vi "Orca Data Spooler Check TL Filename.vi"(0 "Path":path, 11 "Error In":errorcluster) -> (4 "Proof Path":path, 15 "Error Out":errorcluster)   [LabVIEW 2020]
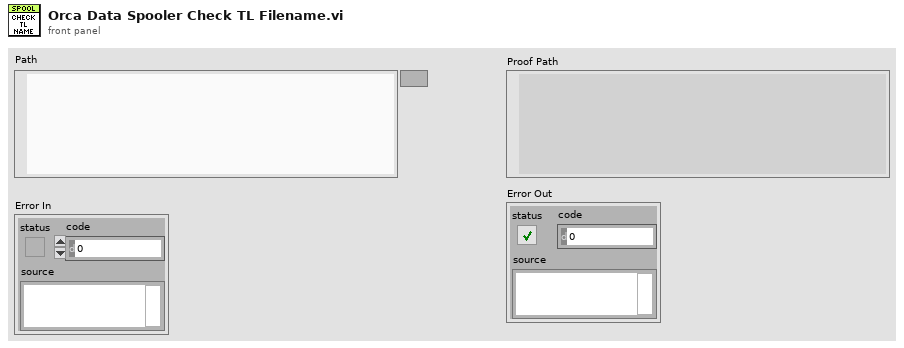
[diagram p1: front panel]
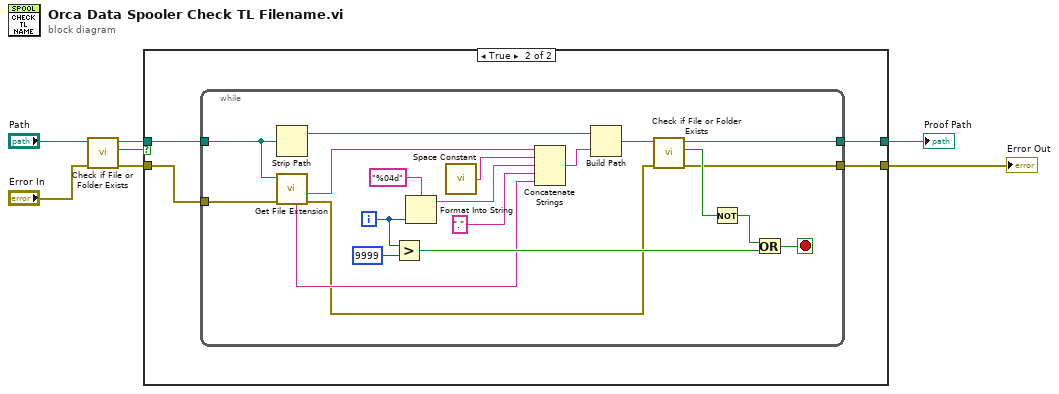
[diagram p0: block diagram]
diagram:
  n1 = call <vilib>:"Check if File or Folder Exists.vi"("error in (no error)"="Error In", "path"="Path") -> ("error out"=w4:errorcluster, "file or folder exists?"=w7:bool, "dup path"=w6:path)  [unwired: 7 in]
  n2 = case shown="True" w7 {
    tunnel: w6 -> [w9 w13]
    tunnel: [w9 w12] -> w5
    tunnel: w4 -> [w8 w10]
    tunnel: [w8 w11] -> w1
    frame False {
    }
    frame True {
      n3 = while {
        tunnel: w13 -> [w19]
        tunnel: [w24] -> w12
        tunnel: [w20] -> w11
        tunnel: w10 -> [w16]
        i -> [w28]
        stop <- w21 stop-if-true
        n4 = Strip Path(path=w19) -> (stripped path=w33:path)  [unwired: 1 out]
        n5 = call <vilib>:"Get File Extension.vi"("error in (no error)"=w16, "file"=w19) -> ("error out"=w14:errorcluster, "filename without extension"=w18:string, "unmodified file extension"=w15:string)  [unwired: 5 in, 2 out]
        n6 = Greater?(x=w28, y=9999) -> (0:w26:bool)
        n7 = Format Into String(format string="%04d", w28) -> (resulting string=w29:string)  [unwired: 2 in, 1 out]
        n8 = call <vilib>:"Space Constant.vi"() -> ("String"=w32:string)
        n9 = Concatenate Strings(w18, w32, w29, ".", w15) -> (w31:string)
        n10 = Build Path(base path=w33, name or relative path=w31) -> (appended path=w25:path)
        n11 = call <vilib>:"Check if File or Folder Exists.vi"("error in (no error)"=w14, "path"=w25) -> ("error out"=w20:errorcluster, "file or folder exists?"=w23:bool, "dup path"=w24:path)  [unwired: 7 in]
        n12 = Not(x=w23) -> (.not. x?=w22:bool)
        n13 = Or(x=w22, y=w26) -> (x .or. y?=w21:bool)
      }
    }
  }
  "Error Out" <- w1
  "Proof Path" <- w5
